vi "AlignString.vi"(7 "min length":i32=12, 10 "Input":string) -> (2 "Output":string)   [LabVIEW 2020, in "Caraya.lvlib" / "Test Report.lvclass"]
uses:
  Test Report/Test Report.lvclass
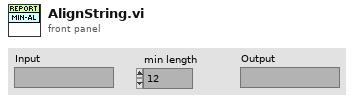
[diagram p1: front panel]
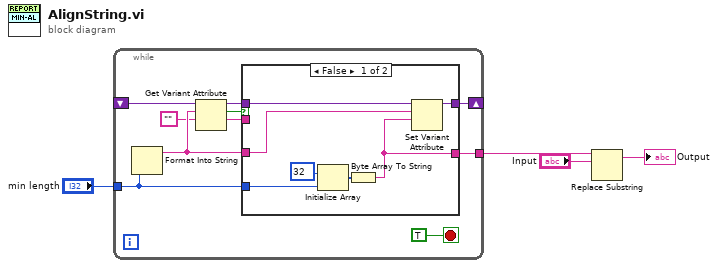
[diagram p0: block diagram]
diagram:
  n1 = while {
    shift-right: [w14] -> _
    shift-left: _ -> [w10]
    tunnel: "min length" -> [w12]
    tunnel: [w11] -> w1
    stop <- TRUE stop-if-true
    n2 = Format Into String(w12) -> (resulting string=w8:string)  [unwired: 3 in, 1 out]
    n3 = Get Variant Attribute(Variant=w10, name=w8, default value (empty Variant)="") -> (duplicate Variant=w9:variant, found=w6:bool, value=w5:string)  [unwired: 1 in, 1 out]
    n4 = case shown="False" w6 {
      tunnel: [w16 w23] -> w14
      tunnel: w9 -> [w19 w23]
      tunnel: w12 -> [w18 _]
      tunnel: [w17 w22] -> w11
      tunnel: w8 -> [w15 _]
      tunnel: w5 -> [_ w22]
      frame False {
        n5 = Initialize Array(u8 32, w18) -> (w21:u8[])
        n6 = Byte Array To String(unsigned byte array=w21) -> (string=w17:string)
        n7 = Set Variant Attribute(Variant=w19, name=w15, value=w17) -> (Variant out=w16:variant)  [unwired: 1 in, 2 out]
      }
      frame True {
      }
    }
  }
  n8 = Replace Substring(4:"Input", 5:w1) -> (1:→"Output":string)  [unwired: 2 in, 1 out]
